vi "Enum Value Change.vi"(7 "tag select":refnum<vi>, 9 "Enum in":refnum<vi>, 10 "dt":i32, 11 "references":T1) -> (0 "error out":errorcluster)   [LabVIEW 2013, in "Table Manager.lvlib"]
uses:
  Table API/Table Manager.lvlib
  object ref.ctl
  tag select module editor node.lvclass
  <vilib>/NI/Tag Bus Data Framework/Configuration Editor/Classes/Engine Parent/Engine Parent Editor Node.lvclass
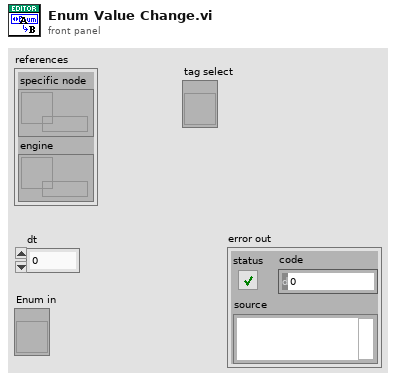
[diagram p1: front panel]
types:
  T1 = typedef "tag select module editor node.lvclass/object ref.ctl" = cluster{"specific node":refnum<data-value>, "engine":refnum<data-value>}
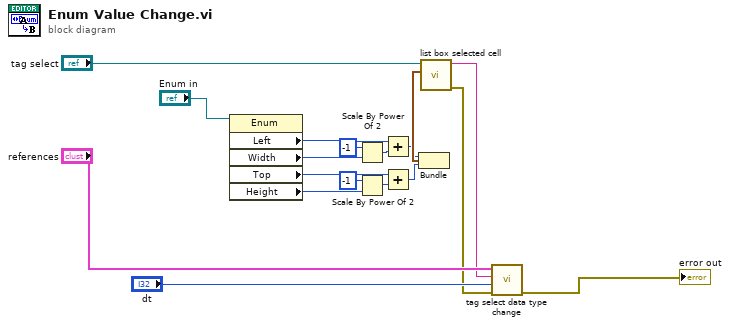
[diagram p0: block diagram]
diagram:
  n1 = property class="Enum"(reference="Enum in") -> ("Left"=w4:i32, "Width"=w1:u32, "Top"=w7:i32, "Height"=w8:u32)  [unwired: 1 in, 2 out]
  n2 = Scale By Power Of 2(n=i16 -1, x=w1) -> (x*2^n=w3:u32)
  n3 = Scale By Power Of 2(n=i16 -1, x=w8) -> (x*2^n=w5:u32)
  n4 = Add(x=w4, y=w3) -> (x+y=w10:u32)
  n5 = Add(x=w7, y=w5) -> (x+y=w9:u32)
  n6 = Bundle(w10, w9) -> (w12:cluster{u32, u32})  [unwired: 1 in]
  n7 = call "list box selected cell.vi"("Coords"=w12, "MulticolumnListbox in"="tag select") -> ("error out"=w15:errorcluster, "tag select name"=w16:string)  [unwired: 6 in, 2 out]
  n8 = call "tag select data type change.vi"("error in"=w15, "Dt Value"="dt", "tag select"=w16, "object ref in"="references") -> ("error out"=→"error out":errorcluster)  [unwired: 6 in, 1 out]
